vi "Request.vi"(8 "error in (no error)":errorcluster, 9 "Device and Axis":string, 10 "Command String":string, 11 "VISA resource name":refnum<visa-resource-name>) -> (0 "error out":errorcluster, 1 "Response Bundle Array":T2(array[cluster]), 2 "Response String Array":string[](array[string]), 3 "VISA resource name out":refnum<visa-resource-name>, 4 "First Response Bundle":T1, 5 "Number of Replies":i32)   [LabVIEW 2015, in "Zaber A Series.lvlib"]
doc: "Writes a string to the serial port and then waits for all of the responses to be received. For inputting the command, it combines the Device and Axis input, Command List input, and Data value input to create a complete command. You could optionally send the complete command directly to the Command List input. Omitting the Device and Axis will send the command to all devices/axes. \n\nYou can use the All Commands or Basic Commands controls for the Command List input to easily select from the list of available commands. For getting or changing settings (get and set commands), you can also use the All Settings and Basic Settings controls as the data input. \n\nThe Enumerate VI is designed to provide an easy list of valid Device and Axis inputs. \n\nAn array containing the complete strings of the responses is returned on the Response String Array output, and the details of the format of the response are described here: http://www.zaber.com/wiki/Manuals/ASCII_Protocol_Manual#Replies. This VI also parses the strings, bundles the components, and returns them as an array of bundles on the Response Bundle Array pin. Additionally a pin returns the number of responses received. \n\nThis VI requires that the Initialize VI has been called with the same serial port."
uses:
  Zaber A Series.lvlib
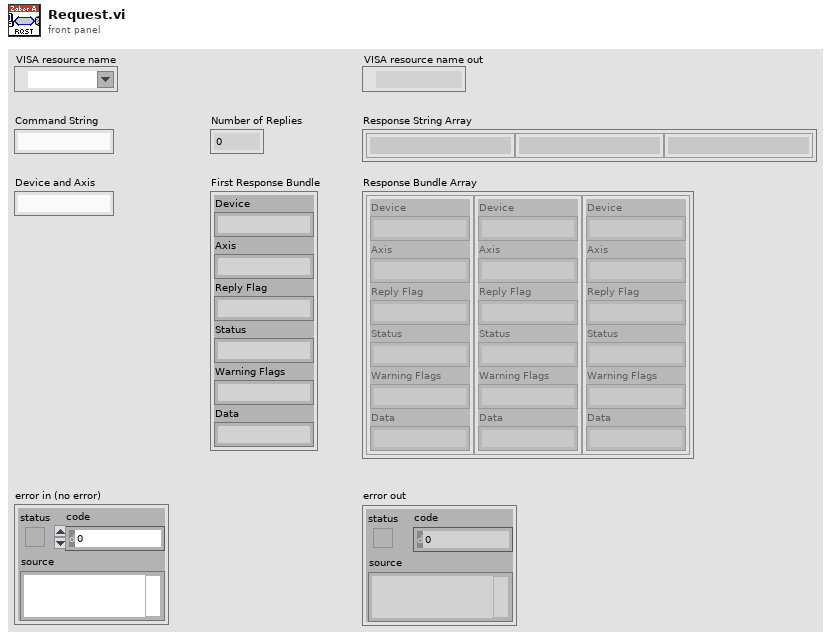
[diagram p1: front panel]
types:
  T1 = cluster{"Device":string, "Axis":string, "Reply Flag":string, "Status":string, "Warning Flags":string, "Data":string}
  T2 = cluster{"Device":string, "Axis":string, "Reply Flag":string, "Status":string, "Warning Flags":string, "Data":string}[]
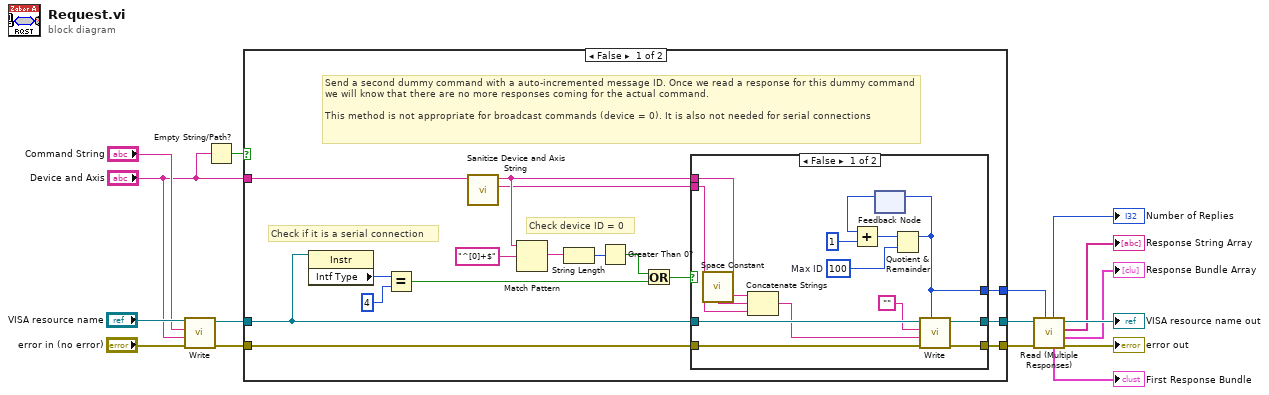
[diagram p0: block diagram]
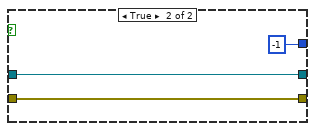
[diagram p2: hidden frame]
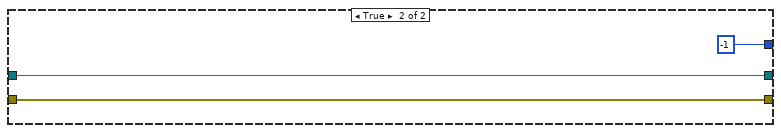
[diagram p3: hidden frame]
diagram:
  n1 = call "Write.vi"("error in (no error)"="error in (no error)", "Device and Axis"="Device and Axis", "Command"="Command String", "VISA resource name"="VISA resource name") -> ("error out"=w7:errorcluster, "VISA resource name out"=w4:refnum<visa-resource-name>)  [unwired: 6 in]
  n2 = Empty String/Path?(string/path="Device and Axis") -> (empty?=w2:bool)
  n3 = case shown="False" w2 {
    tunnel: w7 -> [w32 w51]
    tunnel: [w31 w52] -> w6
    tunnel: [w30 w51] -> w5
    tunnel: w4 -> [w27 w52]
    tunnel: "Device and Axis" -> [w19 _]
    tunnel: [w20 -1] -> w1
    frame False {
      # "Send a second dummy command with a auto-incremented message ID. Once we read a response for this dummy command we will know that there are no more responses coming for the actual command.\n\nThis method is not appropriate for broadcast commands (device = 0). It is also not needed for serial connections"
      # "Check if it is a serial connection"
      # "Check device ID = 0"
      n4 = property class="Instr"(reference=w27) -> ("Intf Type"=w29:u16)  [unwired: 1 in, 2 out]
      n5 = Equal?(x=w29, y=4) -> (x = y?=w22:bool)
      n6 = call "Sanitize Device and Axis String.vi"("Device and Axis"=w19) -> ("Axis Address"=w17:string, "Device Address"=w18:string)  [unwired: 9 in]
      n7 = Match Pattern(string=w18, regular expression="^[0]+$" ("format string")) -> (match substring=w25:string)  [unwired: 1 in, 3 out]
      n8 = String Length(string=w25) -> (length=w24:i32)
      n9 = Greater Than 0?(x=w24) -> (x > 0?=w21:bool)
      n10 = Or(x=w21, y=w22) -> (x .or. y?=w23:bool)
      n11 = case shown="False" w23 {
        tunnel: w27 -> [w42 w49]
        tunnel: w32 -> [w41 w48]
        tunnel: [w40 w49] -> w31
        tunnel: [w39 w48] -> w30
        tunnel: w18 -> [w37 _]
        tunnel: w17 -> [w36 _]
        tunnel: [w33 -1] -> w20
        frame False {
          w43 = 100  # Max ID
          n12 = call <vilib>:"Space Constant.vi"() -> ("String"=w35:string)
          n13 = Concatenate Strings(w37, w35, w36) -> (w34:string)
          n14 = feedback #1() -> (w45:i32)  [unwired: 1 in]
          n15 = Add(x=w45, y=1) -> (x+y=w44:i32)
          n16 = Quotient & Remainder(x=w44, y=w43) -> (x-y*floor(x/y)=w33:i32)  [unwired: 1 out]
          n17 = feedback-in #1(w33) -> ()
          n18 = call "Write.vi"("Message ID (-1)"=w33, "error in (no error)"=w41, "Device and Axis"=w34, "Command"="", "VISA resource name"=w42) -> ("error out"=w39:errorcluster, "VISA resource name out"=w40:refnum<visa-resource-name>)  [unwired: 5 in]
        }
        frame True {
        }
      }
    }
    frame True {
    }
  }
  n19 = call "Read (Multiple Responses).vi"("Termination Message ID (-1)"=w1, "error in (no error)"=w5, "VISA resource name"=w6) -> ("error out"=→"error out":errorcluster, "Response Bundle Array"=→"Response Bundle Array":T2, "Response String Array"=→"Response String Array":string[], "VISA resource name out"=→"VISA resource name out":refnum<visa-resource-name>, "First Response Bundle"=→"First Response Bundle":T1, "Number of Replies"=→"Number of Replies":i32)  [unwired: 3 in]
